vi "PXI8431_com.vi"(10 "Slot":i32=6) -> ()   [LabVIEW 2017]
doc: "Use this template to build a producer/consumer design pattern with events to produce queue items. Use this design pattern instead of the User Interface Event Handler pattern for user interfaces when you want to execute code asynchronously in response to an event without slowing the user interface responsiveness."
uses:
  Hardware/Serial/Serial - Settings.ctl
  controls/FS_PXI8431com.ctl
  controls/FS_PXI8431rs.ctl
  controls/Serial - XON-XOFF Characters.ctl
  controls/Serial - ASCII Characters.ctl
panel:
  in  "Select Port":u16(ring)
  in  "Serial Settings":T1={"baud rate"=9600, "data bits"=8, "parity"=enum."None", "stop bits"=10, "flow control"=0} {"flow control" items=["None"=0, "XON/XOFF"=1, "RTS/CTS"=2, "DTR/DSR"=4]; "stop bits" items=["1.0"=10, "1.5"=15, "2.0"=20]; "data bits" min=5 max=8 step=1; "baud rate" items=["75"=75, "110"=110, "134"=134, "150"=150, "300"=300, "600"=600, "1200"=1200, "1800"=1800, "2400"=2400, "4800"=4800, "7200"=7200, "9600"=9600, "14400"=14400, "19200"=19200, "28800"=28800, "38400"=38400, "56000"=56000, "57600"=57600, "115200"=115200, "128000"=128000, "230400"=230400]}
  in  "OK":bool
  out "数据":string
  in  "命令":string
  # "PXI-8341串口通讯"
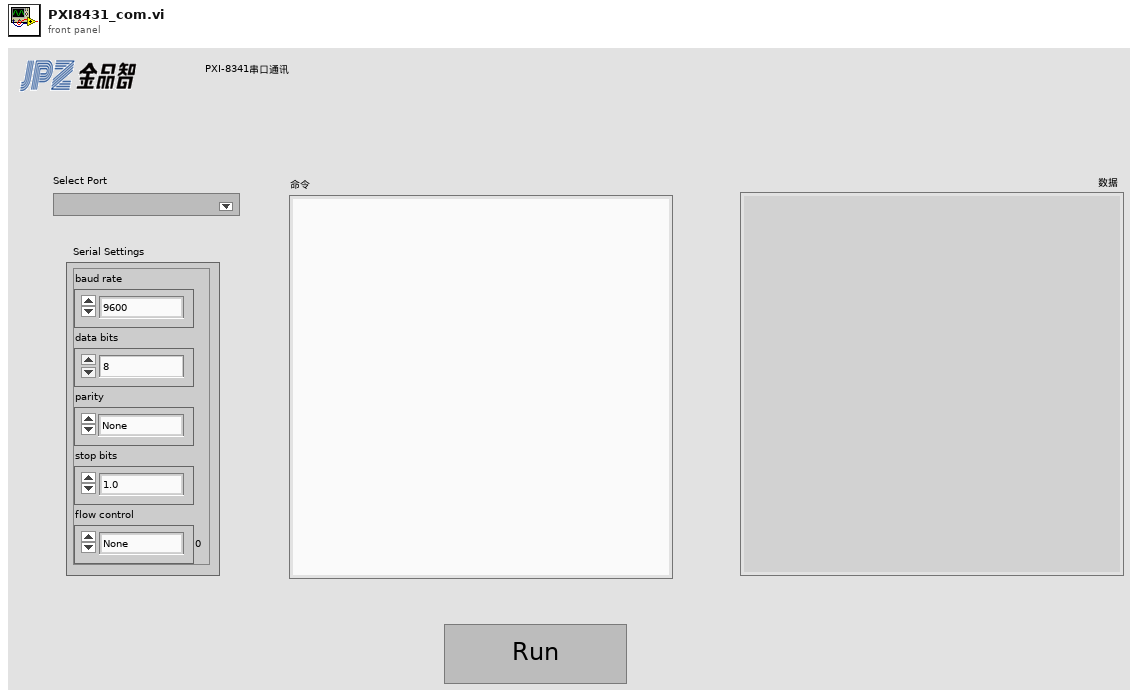
[diagram p1: front panel]
types:
  T1 = typedef "Serial - Settings.ctl" = cluster{"baud rate":u32, "data bits":u16, "parity":enum16{"None", "Odd", "Even", "Mark", "Space"}, "stop bits":u16, "flow control":u16}
  T2 = typedef "FS_PXI8431com.ctl" = enum16{"Initialize", "Select Slot", "Run Com", "Config", "Set Xon/Xoff", "Set TermChar", "Write Command", "Read Data", "Release Port"}
  T3 = typedef "FS_PXI8431rs.ctl" = enum16{"Config Serial", "Xon/Xoff Char", "ASRL TermChar", "Write Command", "Read Data", "Clear Resure"}
  T4 = typedef "Serial - XON-XOFF Characters.ctl" = cluster{"XON":T5, "XOFF":T5}
  T5 = typedef "Serial - ASCII Characters.ctl" = enum16{"NUL", "SOH", "STX", "ETX", "EOT", "ENQ", "ACK", "BEL", "BS", "HT", "LF", "VT", "FF", "CR", "SO", "SI", "DLE", "DC1", "DC2", "DC3", "DC4", "NAK", "SYN", "ETB", "CAN", "EM", "SUB", "ESC", "FS", "GS", "RS", "US", "SP", "!", "\"", "#", "$", "%", "&", "'", "(", ")", "*", "+", ",", "- (-)", ".", "/", "0", "1", "2", "3", "4", "5", "6", "7", "8", "9", ":", ";", "<", "=", ">", "?", "@", "A", "B", "C", "D", "E", "F", "G", "H", "I", "J", "K", "L", "M", "N", "O", "P", "Q", "R", "S", "T", "U", "V", "W", "X", "Y", "Z", "[", "\\", "]", "^", "_", "`", "a", "b", "c", "d", "e", "f", "g", "h", "i", "j", "k", "l", "m", "n", "o", "p", "q", "r", "s", "t", "u", "v", "w", "x", "y", "z", "{", "|", "}", "~"}
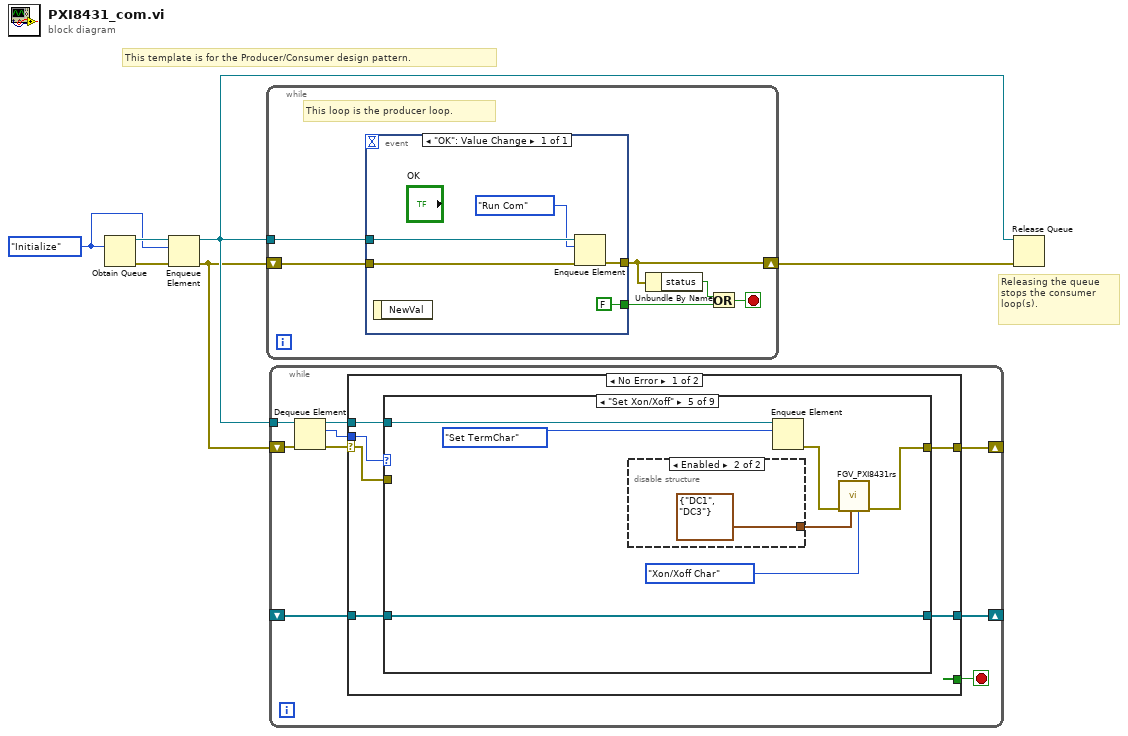
[diagram p0: block diagram]
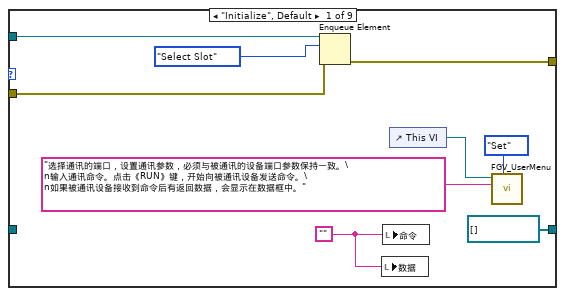
[diagram p2: hidden frame]
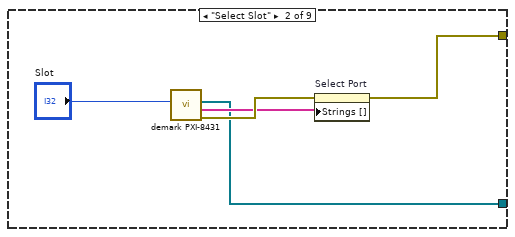
[diagram p3: hidden frame]
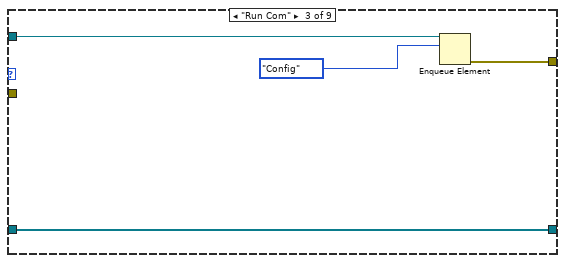
[diagram p4: hidden frame]
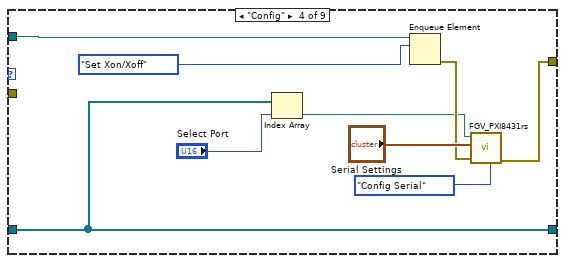
[diagram p5: hidden frame]
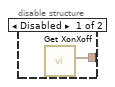
[diagram p6: hidden frame]
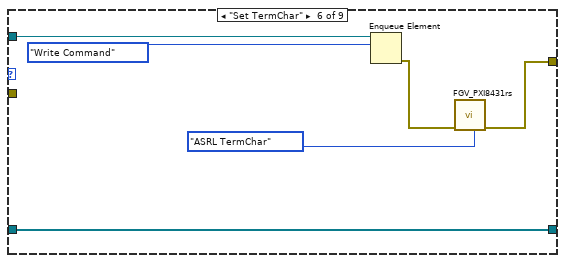
[diagram p7: hidden frame]
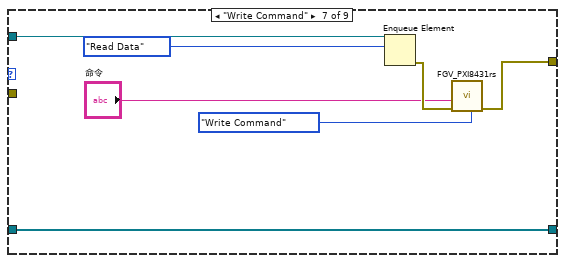
[diagram p8: hidden frame]
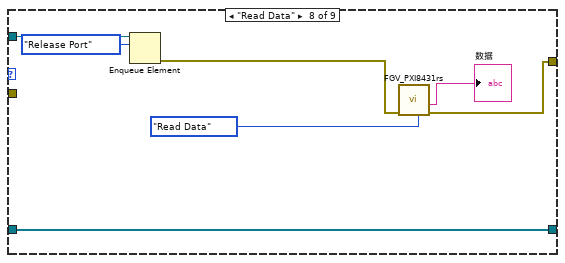
[diagram p9: hidden frame]
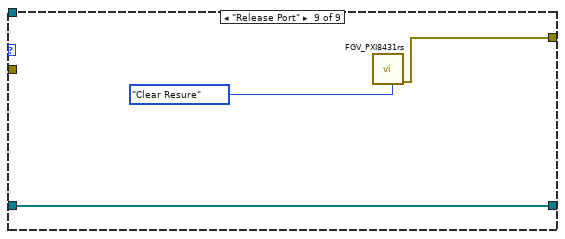
[diagram p10: hidden frame]
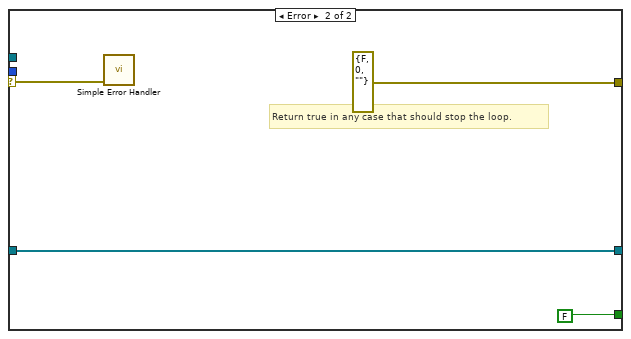
[diagram p11: hidden frame]
diagram:
  w2 = FS_PXI8431com."Initialize"
  # "Releasing the queue stops the consumer loop(s)."
  # "This template is for the Producer/Consumer design pattern."
  n1 = Obtain Queue(element data type=w2) -> (queue out=w5:refnum<queue>, error out=w3:errorcluster)  [unwired: 4 in, 1 out]
  n2 = Enqueue Element(queue=w5, element=w2, error in (no error)=w3) -> (queue out=w4:refnum<queue>, error out=w1:errorcluster)  [unwired: 1 in, 1 out]
  n3 = while {
    shift-right: [w8] -> w6
    shift-left: w1 -> [w11]
    tunnel: w4 -> [w12]
    stop <- w9 stop-if-true
    # "This loop is the producer loop."
    n4 = event shown="[0] \"OK\": Value Change" {
      selector: _ -> [_]
      dyn-events: _ -> [_]
      timeout: _ -> [_]
      tunnel: w12 -> [w17]
      tunnel: w11 -> [w16]
      tunnel: [w15] -> w8
      tunnel: [FALSE ("stop")] -> w10
      event "OK": Value Change {
        n5 = event-data() -> ()  [unwired: 1 in, 1 out]
        n6 = Enqueue Element(queue=w17, element=FS_PXI8431com."Run Com", error in (no error)=w16) -> (error out=w15:errorcluster)  [unwired: 1 in, 2 out]
      }
    }
    n7 = Unbundle By Name(w8) -> ("status"=w7:bool)
    n8 = Or(x=w7, y=w10) -> (x .or. y?=w9:bool)
  }
  n9 = while {
    tunnel: w4 -> [w26]
    shift-right: [w21] -> _
    shift-left: w1 -> [w20]
    shift-right: [w19] -> _
    shift-left: _ -> [w18]
    stop <- w23 stop-if-true
    n10 = Dequeue Element(queue=w26, error in (no error)=w20) -> (queue out=w22:refnum<queue>, element=w24:T2, error out=w25:errorcluster)  [unwired: 1 in, 1 out]
    n11 = case shown="No Error" w25 {
      selector: w25 -> [w27 w93]
      tunnel: w24 -> [w32 _]
      tunnel: [_ FALSE] -> w23
      tunnel: w22 -> [w31 _]
      tunnel: [w30 errorcluster {"status"=FALSE, "code"=0, "source"=""} ("error out")] -> w21
      tunnel: [w29 w92] -> w19
      tunnel: w18 -> [w28 w92]
      frame No Error {
        n12 = case shown="\"Set Xon/Xoff\"" w32 {
          tunnel: w31 -> [w35 _ w50 w58 w66 w74 w81 w88 _]
          tunnel: [w33 w43 w49 w54 w62 w70 w77 w85 w90] -> w30
          tunnel: [refnum<visa-resource-name>[] [] ("VISA Ref") w42 w47 w52 w60 w69 w75 w82 w89] -> w29
          tunnel: w28 -> [_ _ w47 w52 w60 w69 w75 w82 w89]
          tunnel: w27 -> [w34 _ _ _ _ _ _ _ _]
          frame "Initialize", Default {
            w41 = ""
            n13 = Enqueue Element(queue=w35, element=FS_PXI8431com."Select Slot", error in (no error)=w34) -> (error out=w33:errorcluster)  [unwired: 1 in, 2 out]
            n14 = local write "数据"(w41) -> ()
            n15 = local write "命令"(w41) -> ()
            n16 = control-ref of="This VI"() -> (w39:refnum<vi>)
            n17 = call "FGV_UserMenu.vi"("Command"=enum16{"Initialize", "Set", "Get"}."Set", "Use Info"="选择通讯的端口，设置通讯参数，必须与被通讯的设备端口参数保持一致。\n输入通讯命令。点击《RUN》键，开始向被通讯设备发送命令。\n如果被通讯设备接收到命令后有返回数据，会显示在数据框中。", "VI Refnum"=w39) -> ()  [unwired: 8 in, 1 out]
          }
          frame "Select Slot" {
            n18 = call "demark PXI-8431.vi"("Slot"="Slot") -> ("error out"=w45:errorcluster, "COM name"=w44:string[], "VISA Ref"=w42:refnum<visa-resource-name>[])  [unwired: 8 in]
            n19 = property on="Select Port" class="Ring (strict)"(error in=w45, "Strings []"=w44) -> (error out=w43:errorcluster)  [unwired: 1 in, 1 out]
          }
          frame "Run Com" {
            n20 = Enqueue Element(queue=w50, element=FS_PXI8431com."Config") -> (error out=w49:errorcluster)  [unwired: 2 in, 2 out]
          }
          frame "Config" {
            n21 = Index Array(array=w52, index="Select Port") -> (element=w51:refnum<visa-resource-name>)
            n22 = Enqueue Element(queue=w58, element=FS_PXI8431com."Set Xon/Xoff") -> (error out=w55:errorcluster)  [unwired: 2 in, 2 out]
            n23 = call "FGV_PXI8431rs.vi"("Enum"=FS_PXI8431rs."Config Serial", "error in (no error)"=w55, "Serial Settings"="Serial Settings", "VISA resource name"=w51) -> ("error out"=w54:errorcluster)  [unwired: 6 in, 1 out]
          }
          frame "Set Xon/Xoff" {
            n24 = disable-structure shown="Enabled" {
              disable-tunnel: [w67 T4 {"XON"=enum."DC1", "XOFF"=enum."DC3"} ("XON/XOFF Characters")] -> w61
              frame Disabled {
                n25 = call "Get XonXoff.vi"() -> ("Information ou"=w67:T4)  [unwired: 11 in]
              }
              frame Enabled {
              }
            }
            n26 = Enqueue Element(queue=w66, element=FS_PXI8431com."Set TermChar") -> (error out=w64:errorcluster)  [unwired: 2 in, 2 out]
            n27 = call "FGV_PXI8431rs.vi"("Enum"=FS_PXI8431rs."Xon/Xoff Char", "XON/XOFF Characters"=w61, "error in (no error)"=w64) -> ("error out"=w62:errorcluster)  [unwired: 7 in, 1 out]
          }
          frame "Set TermChar" {
            n28 = Enqueue Element(queue=w74, element=FS_PXI8431com."Write Command") -> (error out=w71:errorcluster)  [unwired: 2 in, 2 out]
            n29 = call "FGV_PXI8431rs.vi"("Enum"=FS_PXI8431rs."ASRL TermChar", "error in (no error)"=w71) -> ("error out"=w70:errorcluster)  [unwired: 8 in, 1 out]
          }
          frame "Write Command" {
            n30 = Enqueue Element(queue=w81, element=FS_PXI8431com."Read Data") -> (error out=w79:errorcluster)  [unwired: 2 in, 2 out]
            n31 = call "FGV_PXI8431rs.vi"("Enum"=FS_PXI8431rs."Write Command", "error in (no error)"=w79, "Command"="命令") -> ("error out"=w77:errorcluster)  [unwired: 7 in, 1 out]
          }
          frame "Read Data" {
            n32 = Enqueue Element(queue=w88, element=FS_PXI8431com."Release Port") -> (error out=w86:errorcluster)  [unwired: 2 in, 2 out]
            n33 = call "FGV_PXI8431rs.vi"("Enum"=FS_PXI8431rs."Read Data", "error in (no error)"=w86) -> ("error out"=w85:errorcluster, "Response"=→"数据":string)  [unwired: 8 in]
          }
          frame "Release Port" {
            n34 = call "FGV_PXI8431rs.vi"("Enum"=FS_PXI8431rs."Clear Resure") -> ("error out"=w90:errorcluster)  [unwired: 9 in, 1 out]
          }
        }
      }
      frame Error {
        # "Return true in any case that should stop the loop."
        n35 = call <vilib>:"Simple Error Handler.vi"("error in (no error)"=w93) -> ()  [unwired: 4 in, 5 out]
      }
    }
  }
  n36 = Release Queue(queue=w4, error in (no error)=w6) -> ()  [unwired: 1 in, 3 out]
